vi "电子钢琴.vi"() -> ()   [LabVIEW 2018]
panel:
  out "数值":i16
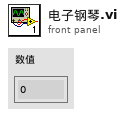
[diagram p1: front panel]
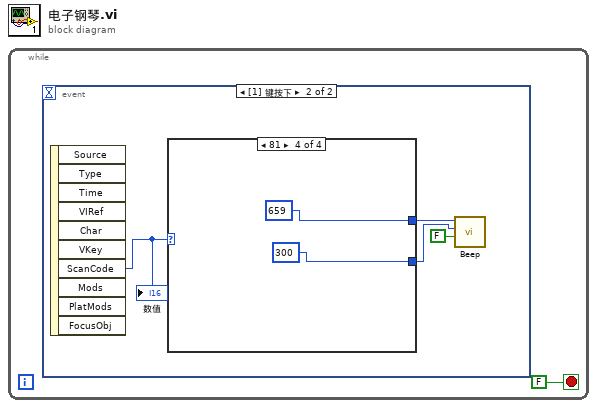
[diagram p0: block diagram]
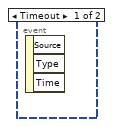
[diagram p2: hidden frame]
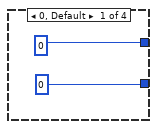
[diagram p3: hidden frame]
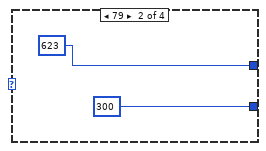
[diagram p4: hidden frame]
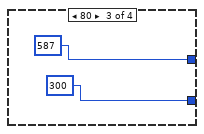
[diagram p5: hidden frame]
diagram:
  n1 = while {
    stop <- FALSE stop-if-true
    n2 = event shown="[1] 键按下" {
      selector: _ -> [_ _]
      dyn-events: _ -> [_ _]
      timeout: _ -> [_ _]
      event Timeout {
        n3 = event-data() -> ()  [unwired: 1 in, 3 out]
      }
      event Key Down {
        n4 = event-data() -> ("ScanCode"=w5:i16)  [unwired: 1 in, 9 out]
        "数值" <- w5
        n5 = case shown="81" w5 {
          tunnel: [0 623 587 659] -> w3
          tunnel: [0 300 300 300] -> w2
          frame 0, Default {
          }
          frame 79 {
          }
          frame 80 {
          }
          frame 81 {
          }
        }
        n6 = call <vilib>:"Beep.vi"("use system alert? (T)"=FALSE, "duration (msec)"=w2, "frequency (Hz)"=w3) -> ()  [unwired: 9 in]
      }
    }
  }
